vi "Main.vi"() -> ()   [LabVIEW 2019, in "CEPM UI.lvlib"]
uses:
  CEPM UI.lvlib
  <vilib>/Utility/error.llb/DialogType.ctl
  <vilib>/SLL Toolkit/SLL Queued State Machine/Queue Driver/Create Queue.vi
  <vilib>/SLL Toolkit/SLL Queued State Machine/Queue Driver/Enqueue an Item to Queue.vi
  <vilib>/SLL Toolkit/SLL Queued State Machine/Queue Driver/Dequeue Queue.vi
  <vilib>/SLL Toolkit/SLL Queued State Machine/Queue Driver/Enqueue N Items.vi
  <vilib>/SLL Toolkit/SLL Queued State Machine/Queue Driver/Flush Queue.vi
  <vilib>/SLL Toolkit/SLL Queued State Machine/Queue Driver/Release Queue.vi
  <vilib>/SLL Toolkit/SLL Queued State Machine/SLL QSM.lvlib
  Core/CEPM.lvlib
  <vilib>/SLL Toolkit/SLL File IO/Spreadsheet/SLL Spreadsheet.lvlib
panel:
  in  "Tab Control":T1(tab)
  in  "Trigger Install":bool
  in  "Trigger Create Copy Exact Package":bool
  out "Create CE Package Status":string
  in  "Reference Package Version (*.csv, Optional)":path
  in  "Package Suffix":string="-CE"
  in  "Existing Package Path":path
  in  "Create":bool
  in  "Install Preview":bool
  in  "Install Package Path":path
  out "Install Status":string
  in  "Install":bool
  out "Install Preview":string
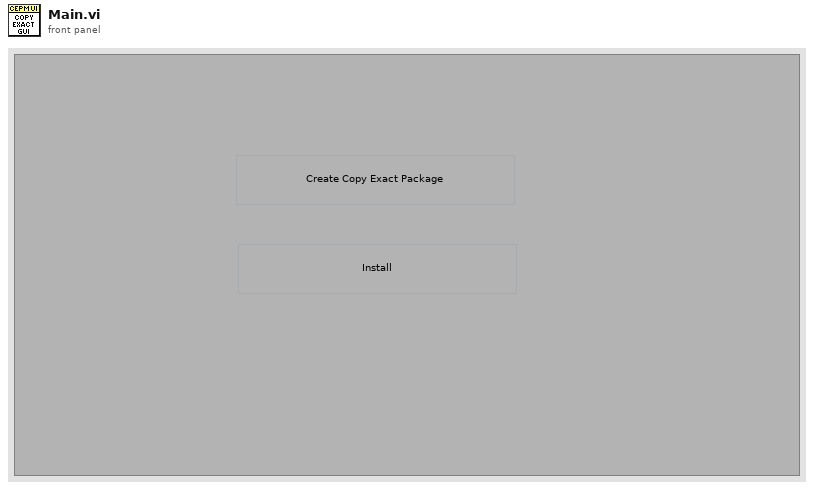
[diagram p1: front panel]
types:
  T1 = enum32{"Starter", "Create Copy Exact Package", "Install Package Inputs", "Install Package"}
  T2 = cluster{"Flags":cluster{"Source Code?":bool}, "Package":string, "Version":string}
  T3 = typedef "DialogType.ctl" = u16
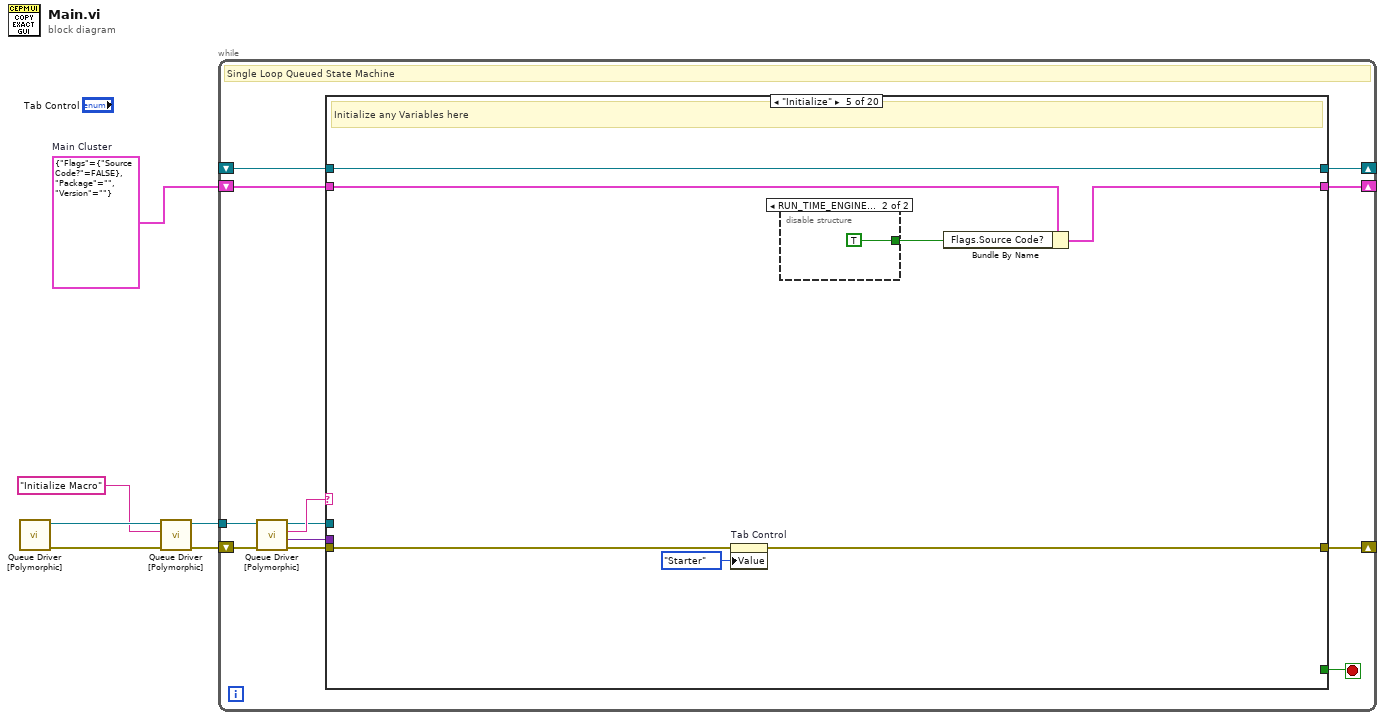
[diagram p0: block diagram]
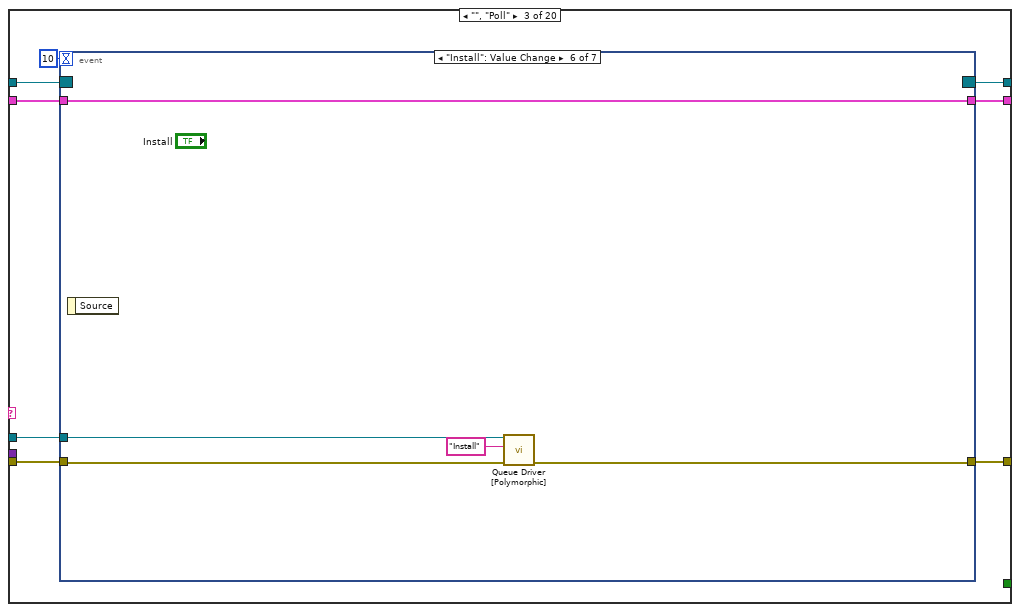
[diagram p4: hidden frame]
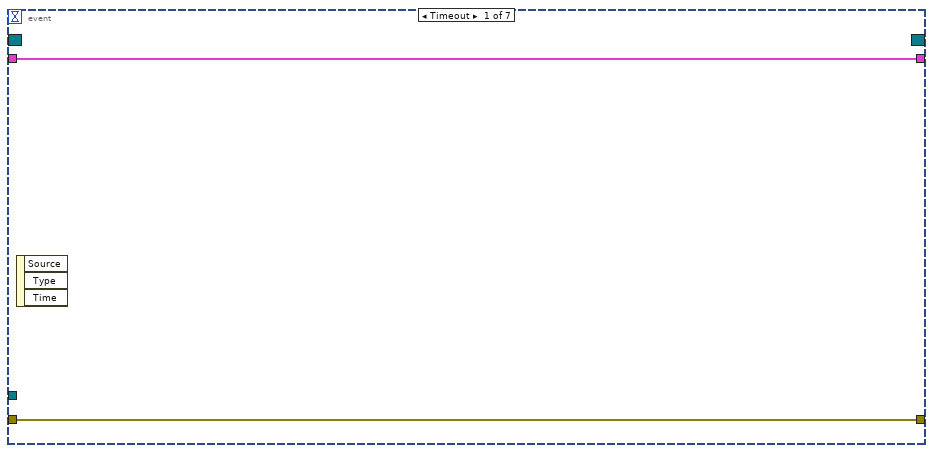
[diagram p5: hidden frame]
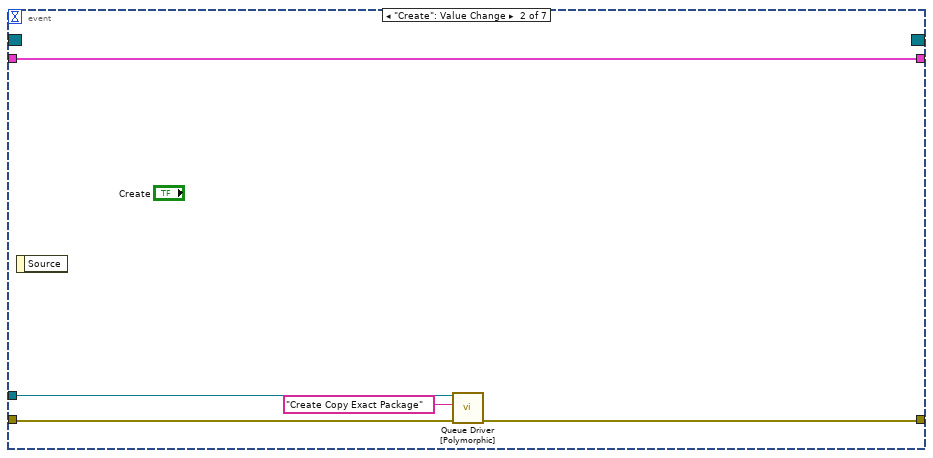
[diagram p6: hidden frame]
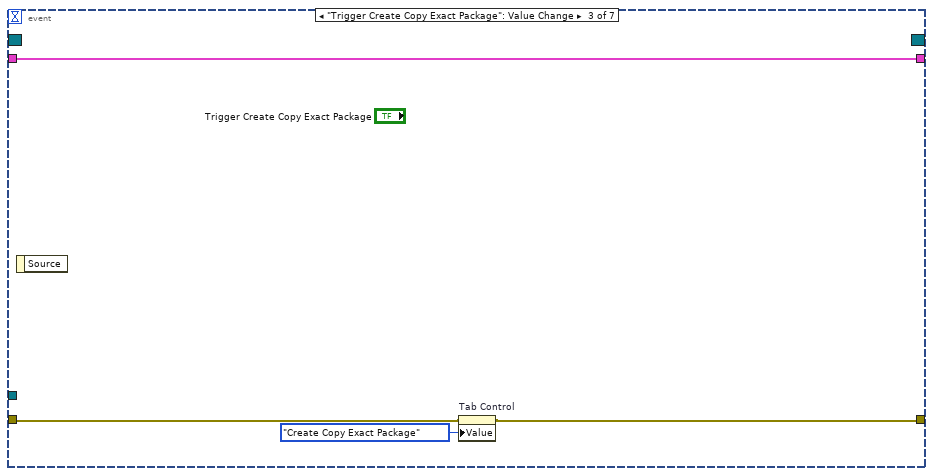
[diagram p7: hidden frame]
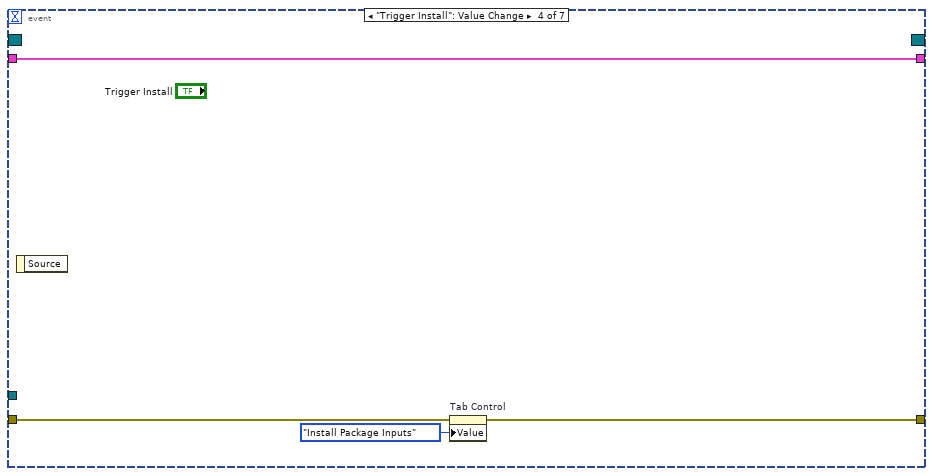
[diagram p8: hidden frame]
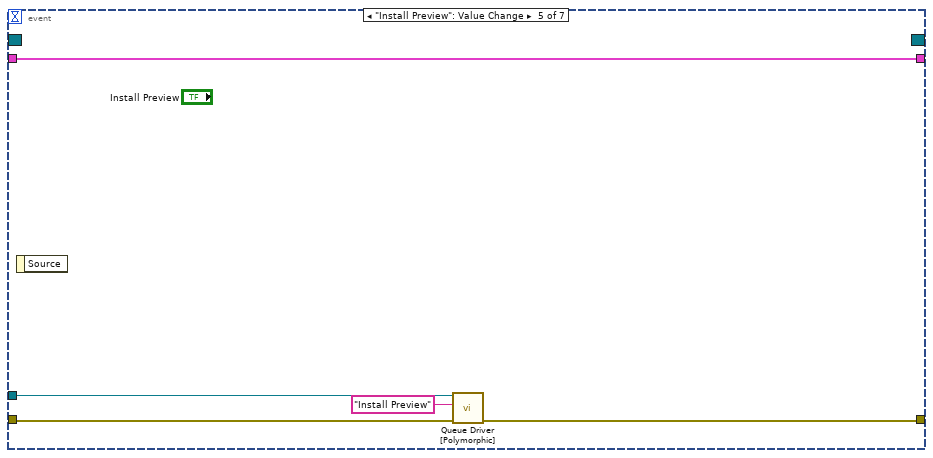
[diagram p9: hidden frame]
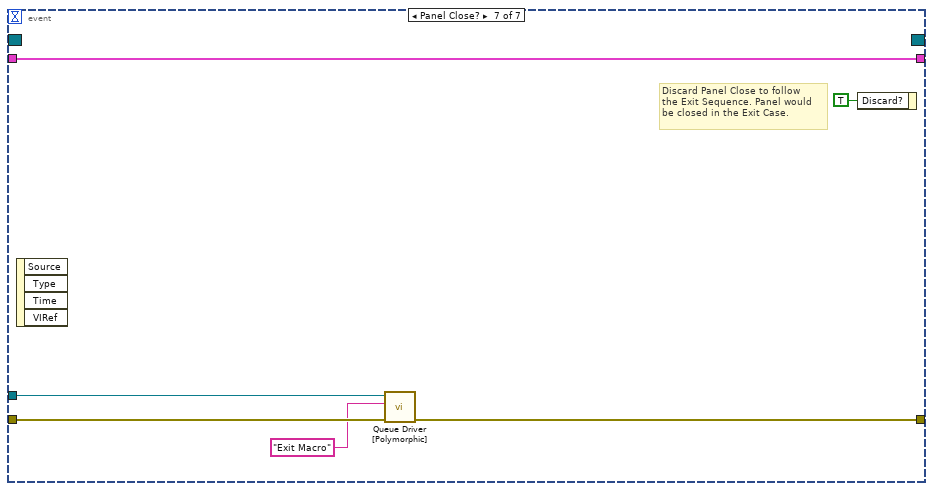
[diagram p10: hidden frame]
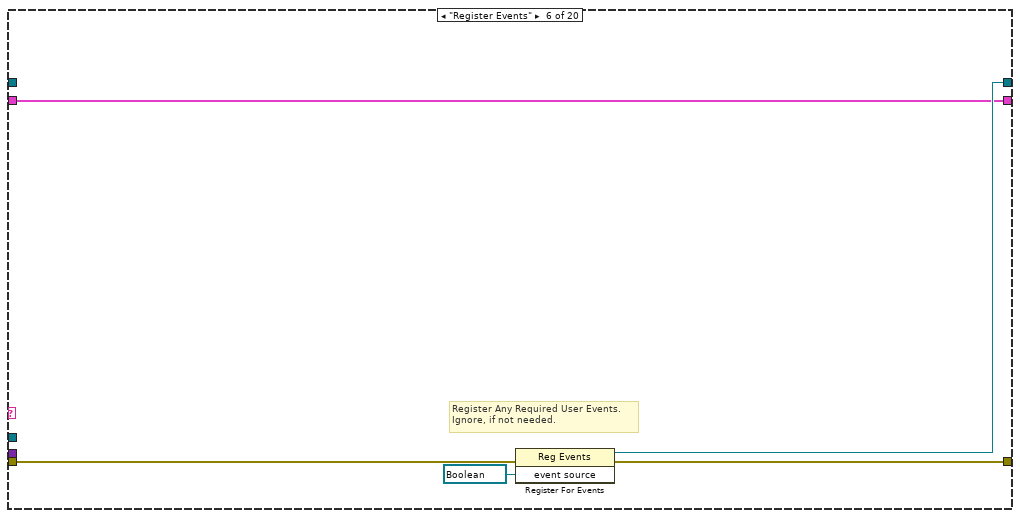
[diagram p13: hidden frame]
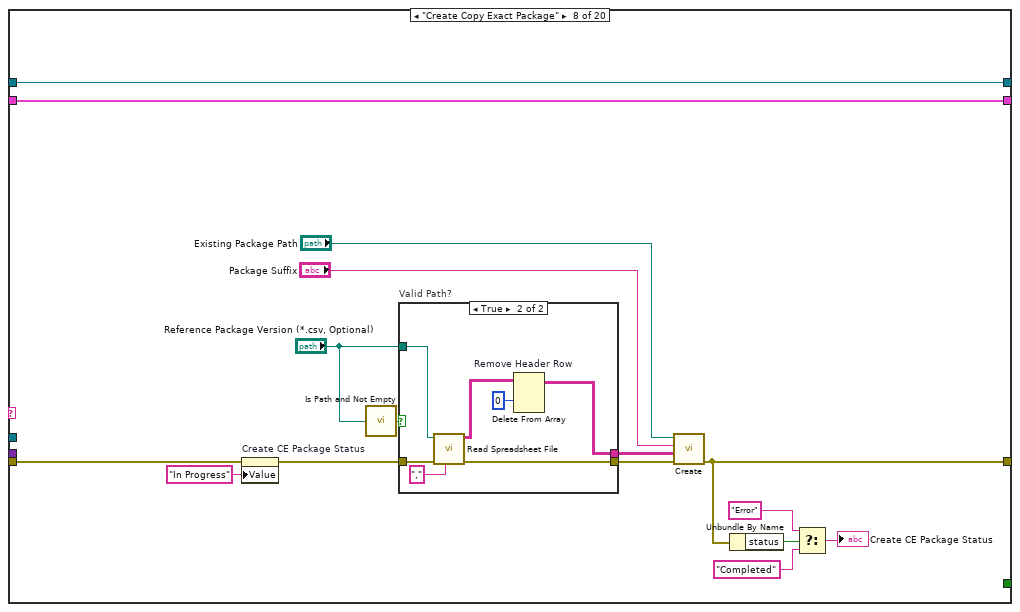
[diagram p15: hidden frame]
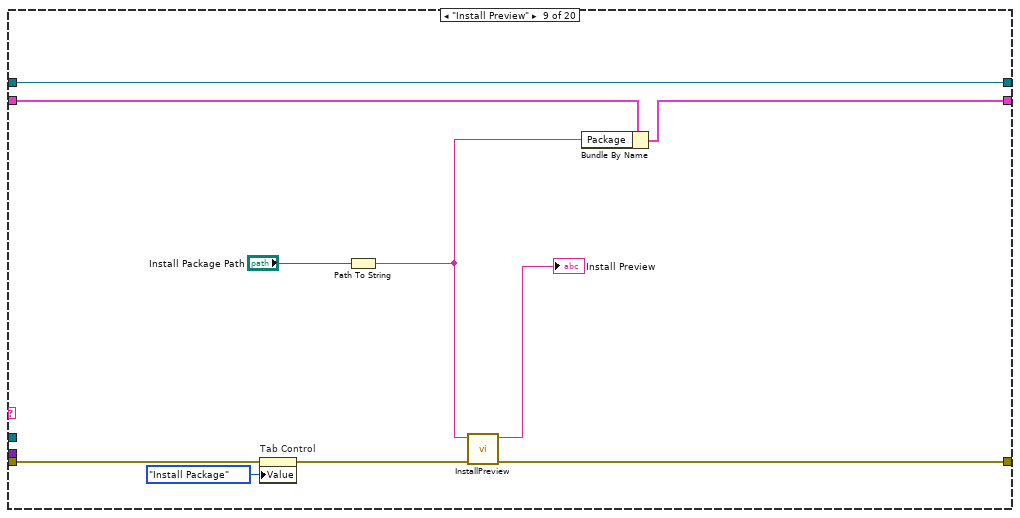
[diagram p17: hidden frame]
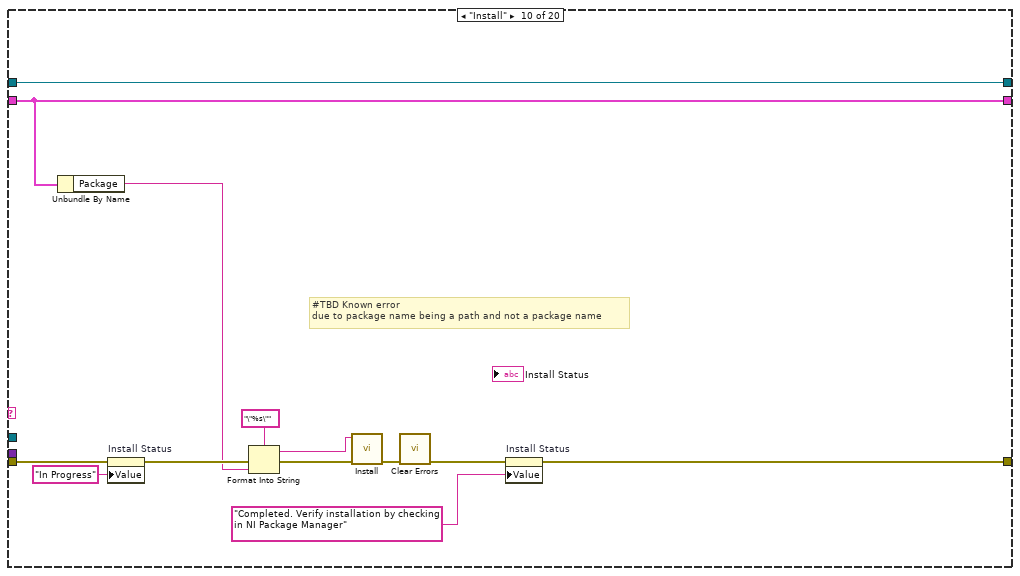
[diagram p18: hidden frame]
diagram:
  w3 = T2 {"Flags"={"Source Code?"=FALSE}, "Package"="", "Version"=""}  # Main Cluster
  n1 = call-poly <vilib>:"Queue Driver [Polymorphic].vi"() -> ("Error Out"=w1:errorcluster, "Queue Ref"=w5:refnum<queue>)  [unwired: 10 in]
  n2 = call-poly <vilib>:"Queue Driver [Polymorphic].vi"("Error In"=w1, "Item to Add"="Initialize Macro", "Queue Ref In"=w5) -> ("Error Out"=w2:errorcluster, "Queue Ref Out"=w6:refnum<queue>)  [unwired: 7 in]
  n3 = while "SLL Queued State Machine" {
    shift-right: [w16] -> _
    shift-left: w2 -> [w18]
    shift-right: [w14] -> _
    shift-left: _ -> [w13]
    shift-right: [w12] -> _
    shift-left: w3 -> [w11]
    tunnel: w6 -> [w9]
    stop <- w15 stop-if-true
    # "Single Loop Queued State Machine"
    n4 = call-poly <vilib>:"Queue Driver [Polymorphic].vi"("Error In"=w18, "Queue Ref In"=w9) -> ("Error Out"=w17:errorcluster, "Data"=w7:variant, "Dequeue"=w10:string, "Queue Ref Out"=w8:refnum<queue>)  [unwired: 6 in]
    n5 = case "QSM Case Structure" shown="\"Initialize\"" w10 {
      selector: w10 -> [_ _ _ _ _ _ _ _ _ _ _ _ _ _ _ _ w154 _ _ _]
      tunnel: w17 -> [w21 w24 w30 w66 w69 w79 w82 w90 w109 w126 w132 w135 w138 w142 w148 w153 w157 w169 w172 w185]
      tunnel: [w21 w24 w31 w66 w68 w78 w82 w87 w114 w118 w132 w135 w138 w141 w147 w153 w160 w167 w172 w181] -> w16
      tunnel: [_ _ _ _ _ _ _ _ _ _ _ _ _ _ _ _ _ _ _ TRUE] -> w15
      tunnel: [w20 w23 w29 w65 w73 w77 w81 w98 w116 w129 w131 w134 w137 w144 w150 w152 w163 w166 w171 w184] -> w14
      tunnel: w13 -> [w20 w23 w28 w65 w73 _ w81 w98 w116 w129 w131 w134 w137 w144 w150 w152 w163 w166 w171 w184]
      tunnel: [w19 w22 w26 w64 w70 w76 w80 w97 w111 w128 w130 w133 w136 w143 w149 w151 w162 w165 w170 w183] -> w12
      tunnel: w11 -> [w19 w22 w27 w64 w71 w76 w80 w97 w115 w128 w130 w133 w136 w143 w149 w151 w162 w165 w170 w183]
      tunnel: w8 -> [_ _ w25 _ _ _ _ _ _ _ _ _ _ w140 w145 _ _ _ _ w174]
      tunnel: w7 -> [_ _ _ _ _ _ _ _ _ _ _ _ _ _ _ _ _ _ _ _]
      frame "/--------------- Read Me -----------------/" {
        # "General Purpose Queue Based State Machine for Any Use Case (main application, module, pop up message etc)\n\nAdvantages:\n1. Lean Project Code Base (dependencies are in vilib).\n2. This template can be safely used in multiple parallel running modules without any issues.\n3. This template can also be safely used even in cases where the VI is configured to be a clone, where multiple \ninstances of the VI could be executing concurrently.\n\nHow to Use:\n1. Add necessary items to the Main Cluster.\n2. Use the Polymorphic Queue Driver for doing any queue operations. \n3. Add any required user events in the \"Register Events\" case. Ignore if not needed.\n4. Use \"Macros\" section for defining any list of state calls, which could be used in multiple places. \nEx: Initialize Macro, might be needed if we need to any reinitialization."
      }
      frame "/------------------ Poll -------------------/" {
      }
      frame "", "Poll" {
        n6 = event shown="[5] \"Install\": Value Change" {
          selector: w28 -> [_ _ _ _ _ _ _]
          dyn-events: [_ _ _ _ _ _ _] -> w29
          timeout: 10 -> [_ _ _ _ _ _ _]
          tunnel: [w34 w35 w41 w45 w48 w53 w62] -> w31
          tunnel: w30 -> [w34 w38 w42 w46 w51 w56 w63]
          tunnel: w27 -> [w33 w39 w43 w47 w52 w57 w61]
          tunnel: [w33 w39 w43 w47 w52 w57 w61] -> w26
          tunnel: w25 -> [_ w37 _ _ w50 w55 w59]
          event Timeout {
            n7 = event-data() -> ()  [unwired: 1 in, 3 out]
          }
          event "Create": Value Change {
            n8 = event-data() -> ()  [unwired: 1 in, 1 out]
            n9 = call-poly <vilib>:"Queue Driver [Polymorphic].vi"("Error In"=w38, "Item to Add"="Create Copy Exact Package", "Queue Ref In"=w37) -> ("Error Out"=w35:errorcluster)  [unwired: 7 in, 1 out]
          }
          event "Trigger Create Copy Exact Package": Value Change {
            n10 = event-data() -> ()  [unwired: 1 in, 1 out]
            n11 = property on="Tab Control" class="TabCtl (strict)"(error in=w42, "Value"=T1."Create Copy Exact Package" ("Tab Control")) -> (error out=w41:errorcluster)  [unwired: 1 in, 1 out]
          }
          event "Trigger Install": Value Change {
            n12 = event-data() -> ()  [unwired: 1 in, 1 out]
            n13 = property on="Tab Control" class="TabCtl (strict)"(error in=w46, "Value"=T1."Install Package Inputs" ("Tab Control")) -> (error out=w45:errorcluster)  [unwired: 1 in, 1 out]
          }
          event "Install Preview": Value Change {
            n14 = event-data() -> ()  [unwired: 1 in, 1 out]
            n15 = call-poly <vilib>:"Queue Driver [Polymorphic].vi"("Error In"=w51, "Item to Add"="Install Preview", "Queue Ref In"=w50) -> ("Error Out"=w48:errorcluster)  [unwired: 7 in, 1 out]
          }
          event "Install": Value Change {
            n16 = event-data() -> ()  [unwired: 1 in, 1 out]
            n17 = call-poly <vilib>:"Queue Driver [Polymorphic].vi"("Error In"=w56, "Item to Add"="Install", "Queue Ref In"=w55) -> ("Error Out"=w53:errorcluster)  [unwired: 7 in, 1 out]
          }
          event Panel Close? {
            # "Discard Panel Close to follow\nthe Exit Sequence. Panel would\nbe closed in the Exit Case."
            n18 = event-data() -> ()  [unwired: 1 in, 4 out]
            n19 = call-poly <vilib>:"Queue Driver [Polymorphic].vi"("Error In"=w63, "Item to Add"="Exit Macro" ("Enqueue"), "Queue Ref In"=w59) -> ("Error Out"=w62:errorcluster)  [unwired: 7 in, 1 out]
            n20 = event-data("Discard?"=TRUE) -> ()  [unwired: 1 in, 1 out]
          }
        }
      }
      frame "/--------------- Initialize -----------------/" {
      }
      frame "Initialize" {
        # "Initialize any Variables here"
        n21 = property on="Tab Control" class="TabCtl (strict)"(error in=w69, "Value"=T1."Starter" ("Tab Control")) -> (error out=w68:errorcluster)  [unwired: 1 in, 1 out]
        n22 = disable-structure shown="RUN_TIME_ENGINE==False" {
          disable-tunnel: [_ TRUE] -> w72
          frame condition #0 {
          }
          frame condition #1 (active) {
          }
        }
        n23 = Bundle By Name(cluster=w71, "Flags.Source Code?"=w72) -> (w70:T2)
      }
      frame "Register Events" {
        # "Register Any Required User Events. \nIgnore, if not needed."
        n24 = register-events(error in=w79, refnum<vi> refnum ("event source")) -> (reference out=w77:refnum<event-registration>, error out=w78:errorcluster)  [unwired: 1 in]
      }
      frame "/---------- Custom Case Splitter ----------/" {
      }
      frame "Create Copy Exact Package" {
        n25 = property on="Create CE Package Status" class="Str"(error in=w90, "Value"="In Progress" ("Create CE Package Status")) -> (error out=w89:errorcluster)  [unwired: 1 in, 1 out]
        n26 = call <vilib>:"Is Path and Not Empty.vi"("path"="Reference Package Version (*.csv, Optional)") -> ("Is Path and Not Empty?"=w91:bool)  [unwired: 4 in]
        n27 = case "Valid Path?" shown="True" w91 {
          tunnel: [w99 w106] -> w94
          tunnel: [_ w100] -> w93
          tunnel: "Reference Package Version (*.csv, Optional)" -> [_ w105]
          tunnel: w89 -> [w99 w104]
          frame False {
          }
          frame True {
            n28 = call <vilib>:"Read Spreadsheet File.vi"("Delimiter (tab)"=",", "error in (no error)"=w104, "File Path"=w105) -> ("error out"=w106:errorcluster, "2D Array"=w102:string[][])  [unwired: 7 in]
            n29 = Delete From Array "Remove Header Row"(array=w102, index (row)=0) -> (array with subset deleted=w100:string[][])  [unwired: 2 in, 1 out]
          }
        }
        n30 = call "Create.vi"("Error In"=w94, "Reference Package Versions (Optional)"=w93, "Package Suffix"="Package Suffix", "Package Path"="Existing Package Path") -> ("Error Out"=w87:errorcluster)  [unwired: 7 in]
        n31 = Unbundle By Name(w87) -> ("status"=w86:bool)
        n32 = Select(t="Error", s=w86, f="Completed") -> (s? t:f=→"Create CE Package Status":string)
      }
      frame "Install Preview" {
        n33 = property on="Tab Control" class="TabCtl (strict)"(error in=w109, "Value"=T1."Install Package" ("Tab Control")) -> (error out=w108:errorcluster)  [unwired: 1 in, 1 out]
        n34 = Path To String(path="Install Package Path") -> (string=w110:string)
        n35 = call "InstallPreview.vi"("Error In"=w108, "Package Name"=w110) -> ("Error Out"=w114:errorcluster, "Preview"=→"Install Preview":string)  [unwired: 8 in]
        n36 = Bundle By Name(cluster=w115, "Package"=w110) -> (w111:T2)
      }
      frame "Install" {
        # "#TBD Known error\ndue to package name being a path and not a package name"
        n37 = Unbundle By Name(w128) -> ("Package"=w122:string)
        n38 = property on="Install Status" class="Str"(error in=w126, "Value"="In Progress" ("Install Status")) -> (error out=w125:errorcluster)  [unwired: 1 in, 1 out]
        n39 = Format Into String(format string="\"%s\"", error in=w125, w122) -> (resulting string=w123:string, error out=w124:errorcluster)  [unwired: 1 in]
        n40 = call "Install.vi"("Error In"=w124, "Package Name"=w123) -> ("Error Out"=w127:errorcluster)  [unwired: 8 in, 1 out]
        n41 = call <vilib>:"Clear Errors.vi"("error in (no error)"=w127) -> ("error out"=w119:errorcluster)  [unwired: 5 in, 1 out]
        n42 = property on="Install Status" class="Str"(error in=w119, "Value"="Completed. Verify installation by checking in NI Package Manager" ("Install Status")) -> (error out=w118:errorcluster)  [unwired: 1 in, 1 out]
      }
      frame "/-------------- User Interface --------------/" {
        # "Duplicate this case to create additional case splitters for readability"
      }
      frame "Update UI" {
        # "Update Front Panel Controls in this Case"
      }
      frame "/----------------- Macros -----------------/" {
      }
      frame "Initialize Macro" {
        w139 = string[] ["Initialize", "Register Events", "Update UI"]  # Initialize Macro
        n43 = call-poly <vilib>:"Queue Driver [Polymorphic].vi"("Error In"=w142, "Enqueue N"=w139, "Queue Ref In"=w140) -> ("Error Out"=w141:errorcluster)  [unwired: 7 in, 1 out]
      }
      frame "Exit Macro" {
        n44 = call-poly <vilib>:"Queue Driver [Polymorphic].vi"("Error In"=w148, "Enqueue N"=string[] ["Exit"], "Queue Ref In"=w145) -> ("Error Out"=w147:errorcluster)  [unwired: 7 in, 1 out]
      }
      frame "/-------------- Error Handler--------------/" {
      }
      frame Default {
        # "Undefined Case/Spelling Errors - Show Message to Developer"
        n45 = property class="VI"(error in=w157) -> (error out=w156:errorcluster, "Name"=w155:string)  [unwired: 1 in, 1 out]
        n46 = Format Into String(format string="\"%s\" in the VI - %s" ("message"), initial string="Undefined case - ", error in=w156, w154, w155) -> (resulting string=w158:string, error out=w160:errorcluster)
        n47 = One Button Dialog(message=w158) -> ()  [unwired: 1 in, 1 out]
      }
      frame "Error" {
        w164 = T3 2 items=["no dialog", "OK message", "continue or stop message", "OK message + warnings", "continue/stop + warnings"] ("type of dialog (OK msg:1)")
        # "Handle the Error"
        n48 = call <vilib>:"Simple Error Handler.vi"("type of dialog (OK msg:1)"=w164, "error in (no error)"=w169) -> ("error out"=w168:errorcluster)  [unwired: 3 in, 4 out]
        n49 = call <vilib>:"Clear Errors.vi"("error in (no error)"=w168) -> ("error out"=w167:errorcluster)  [unwired: 5 in, 1 out]
      }
      frame "/------------------- Exit --------------------/" {
      }
      frame "Exit" {
        n50 = call-poly <vilib>:"Queue Driver [Polymorphic].vi"("Error In"=w185, "Queue Ref In"=w174) -> ("Error Out"=w186:errorcluster, "Queue Ref Out"=w173:refnum<queue>)  [unwired: 7 in, 1 out]
        n51 = Unbundle By Name(w183) -> ("Flags.Source Code?"=w176:bool)
        n52 = call-poly <vilib>:"Queue Driver [Polymorphic].vi"("Error In"=w186, "Queue Ref In"=w173) -> ("Error Out"=w182:errorcluster)  [unwired: 9 in]
        n53 = Call Chain() -> (call chain=w180:string[])
        n54 = Array Size(array=w180) -> (size(s)=w179:i32)
        n55 = Equal?(x=w179, y=1) -> (x = y?=w177:bool)
        n56 = And(x=w176, y=w177) -> (x .and. y?=w175:bool)
        n57 = case "Skip Panel Close when in Source\nCode and is the top most caller" shown="False" w175 {
          tunnel: w182 -> [w189 w191]
          tunnel: [w190 w191] -> w181
          frame False {
            # "Close Panel"
            n58 = invoke class="VI" method="FP.Close"() -> (error out=w188:errorcluster)  [unwired: 3 in, 2 out]
            n59 = Merge Errors(w189, w188) -> (w190:errorcluster)
          }
          frame True {
            # "Do Not Close Panel"
          }
        }
      }
    }
  }
